vi "L298N.vi"(4 "Turn Off":bool, 5 "IN 4":u8, 6 "PWM Channel":u8, 7 "IN3":u8, 8 "Error In":errorcluster, 9 "Source Voltage":dbl(knob) scale=0.0..10.0, 10 "Voltage":dbl(knob) scale=0.0..10.0, 11 "LINX Resource IN":T1) -> (0 "Error Out":errorcluster, 3 "LINX Resource OUT":T1)   [LabVIEW 2016]
uses:
  <vilib>/MakerHub/LINX/Private/Type Defs/LINX Ref.ctl
  <vilib>/MakerHub/LINX/Private/Type Defs/Platform.ctl
  <vilib>/MakerHub/LINX/Private/Type Defs/Interface.ctl
  <vilib>/MakerHub/LINX/Private/Device/Type Defs/LINX Device Config.ctl
  <vilib>/MakerHub/LINX/Private/Device/Type Defs/TCP Config.ctl
  <vilib>/MakerHub/LINX/Private/Device/Type Defs/Channels.ctl
  <vilib>/MakerHub/LINX/Public/Peripherals/Digital/Digital Write 1 Chan.vi
  <vilib>/MakerHub/LINX/Public/Peripherals/PWM/PWM Set Duty Cycle 1 Chan.vi
  <vilib>/MakerHub/LINX/Public/Peripherals/Digital/Digital Write N Chans.vi
  <vilib>/MakerHub/LINX/Private/Local IO/LinxDigitalWrite.vi
  <vilib>/MakerHub/LINX/Public/Utilities/Check Channel.vi
  <vilib>/MakerHub/LINX/Private/Utilties/Generate Error.vi
  <vilib>/MakerHub/LINX/Public/Peripherals/PWM/PWM Set Duty Cycle N Chans.vi
  <vilib>/MakerHub/LINX/LMH-LINX.lvlib
  <vilib>/MakerHub/LINX/Private/Device/Device.lvlib
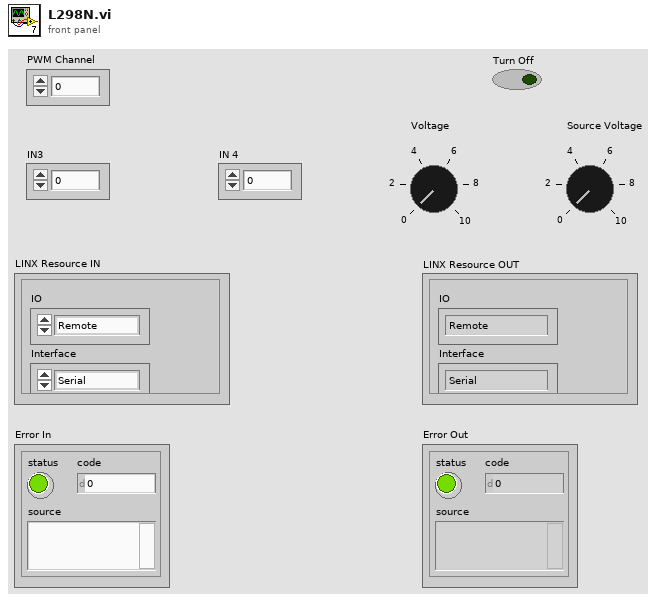
[diagram p1: front panel]
types:
  T1 = typedef "LMH-LINX.lvlib/LINX Ref.ctl" = cluster{"IO":T2, "Interface":T3, "LINX Device Config":T4}
  T2 = typedef "LMH-LINX.lvlib/Platform.ctl" = enum16{"Remote", "Local"}
  T3 = typedef "LMH-LINX.lvlib/Interface.ctl" = enum16{"Serial", "TCP"}
  T4 = typedef "LMH-LINX.lvlib/Device.lvlib/LINX Device Config.ctl" = cluster{"Interface":T3, "COM Port":refnum<visa-resource-name>, "TCP Configuration":T5, "Device Family":u8, "Device ID":u8, "Device Name":string, "TCP Ref":refnum<k5>, "Channels":T6}
  T5 = typedef "LMH-LINX.lvlib/Device.lvlib/TCP Config.ctl" = cluster{"IP Address":string, "Port":u16}
  T6 = typedef "LMH-LINX.lvlib/Channels.ctl" = cluster{"DI":u8[], "DO":u8[], "AI":u8[], "AO":u8[], "PWM":u8[], "QE":u8[], "UART":u8[], "I2C 2":u8[], "SPI":u8[], "CAN":u8[], "Servo":u8[], "AI Ref (V)":dbl, "AI Resolution (Bits)":u8, "AO Ref (V)":dbl, "AO Resolution (Bits)":u8}
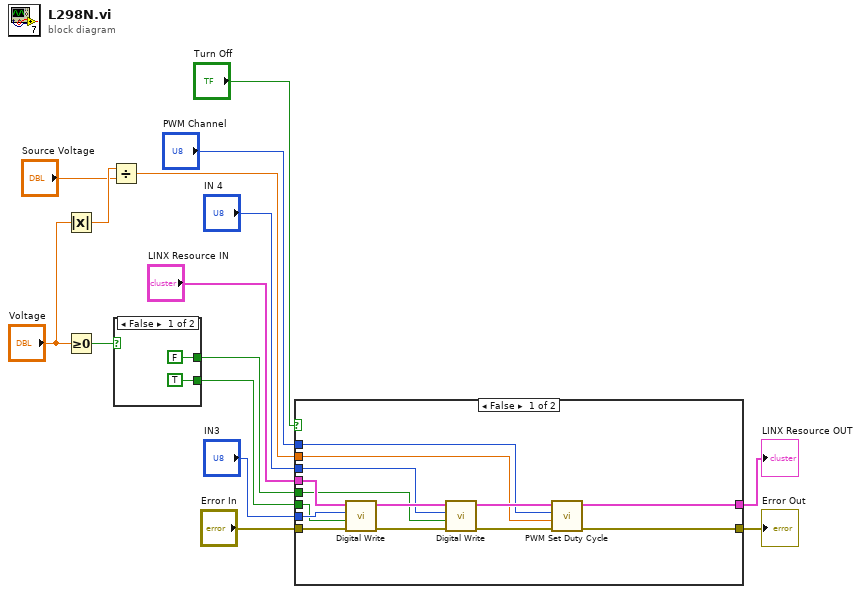
[diagram p0: block diagram]
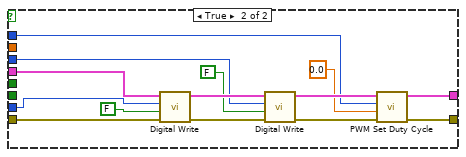
[diagram p2: hidden frame]
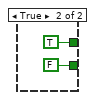
[diagram p3: hidden frame]
diagram:
  n1 = Absolute Value(x="Voltage") -> (abs(x)=w14:dbl)
  n2 = Greater Or Equal To 0?(x="Voltage") -> (x >= 0?=w12:bool)
  n3 = Divide(x=w14, y="Source Voltage") -> (x/y=w3:dbl)
  n4 = case shown="False" w12 {
    tunnel: [FALSE TRUE] -> w2
    tunnel: [TRUE FALSE] -> w1
    frame False {
    }
    frame True {
    }
  }
  n5 = case shown="False" "Turn Off" {
    tunnel: "IN3" -> [w29 w41]
    tunnel: "LINX Resource IN" -> [w28 w43]
    tunnel: "Error In" -> [w27 w42]
    tunnel: [w26 w38] -> w7
    tunnel: [w25 w37] -> w6
    tunnel: "IN 4" -> [w24 w40]
    tunnel: "PWM Channel" -> [w23 w39]
    tunnel: w3 -> [w22 _]
    tunnel: w2 -> [w21 _]
    tunnel: w1 -> [w20 _]
    frame False {
      n6 = call-poly <vilib>:"Digital Write.vi"("Error In"=w27, "Output Value"=w20, "DO Channel"=w29, "LINX Resource"=w28) -> ("Error Out"=w32:errorcluster, "LINX Resource"=w33:T1)  [unwired: 6 in]
      n7 = call-poly <vilib>:"Digital Write.vi"("Error In"=w32, "Output Value"=w21, "DO Channel"=w24, "LINX Resource"=w33) -> ("Error Out"=w30:errorcluster, "LINX Resource"=w31:T1)  [unwired: 6 in]
      n8 = call-poly <vilib>:"PWM Set Duty Cycle.vi"("Error In"=w30, "Duty Cycle (0-1)"=w22, "PWM Channel"=w23, "LINX Resource"=w31) -> ("Error Out"=w25:errorcluster, "LINX Resource"=w26:T1)  [unwired: 6 in]
    }
    frame True {
      n9 = call-poly <vilib>:"Digital Write.vi"("Error In"=w42, "Output Value"=FALSE, "DO Channel"=w41, "LINX Resource"=w43) -> ("Error Out"=w46:errorcluster, "LINX Resource"=w47:T1)  [unwired: 6 in]
      n10 = call-poly <vilib>:"Digital Write.vi"("Error In"=w46, "Output Value"=FALSE, "DO Channel"=w40, "LINX Resource"=w47) -> ("Error Out"=w44:errorcluster, "LINX Resource"=w45:T1)  [unwired: 6 in]
      n11 = call-poly <vilib>:"PWM Set Duty Cycle.vi"("Error In"=w44, "Duty Cycle (0-1)"=0.0, "PWM Channel"=w39, "LINX Resource"=w45) -> ("Error Out"=w37:errorcluster, "LINX Resource"=w38:T1)  [unwired: 6 in]
    }
  }
  "LINX Resource OUT" <- w7
  "Error Out" <- w6
